vi "IMAQ Name Create.vi"(8 "error in (no error)":errorcluster, 10 "Name (\"\")":string, 11 "Video File in":refnum<class "Video File.lvclass">) -> (0 "error out":errorcluster, 2 "Name Out":string, 3 "Video File out":refnum<class "Video File.lvclass">)   [LabVIEW 2018, in "Video File.lvclass"]
uses:
  Video File.lvclass
  Video File.lvclass/Video File.ctl
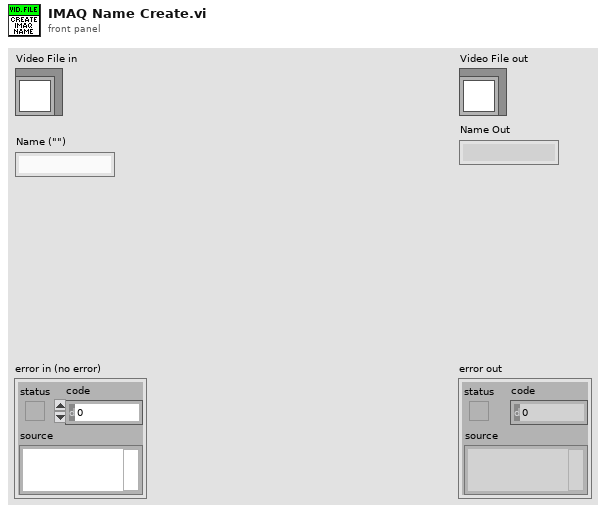
[diagram p1: front panel]
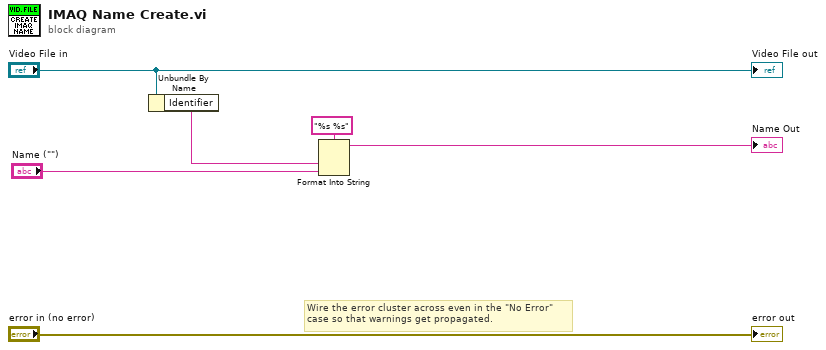
[diagram p0: block diagram]
diagram:
  # "Wire the error cluster across even in the \"No Error\"\ncase so that warnings get propagated."
  n1 = Unbundle By Name("Video File in") -> ("Identifier"=w1:string)
  n2 = Format Into String(format string="%s %s", w1, "Name (\"\")") -> (resulting string=→"Name Out":string)  [unwired: 2 in, 1 out]
  "error out" <- "error in (no error)"
  "Video File out" <- "Video File in"
